vi "Flatten (single).vi"(8 "error in (no error)":errorcluster, 9 "y (0)":dbl, 10 "x (0)":dbl, 11 "XY-data":cluster{"X-array":dbl[], "Y-array":dbl[]}) -> (0 "error out":errorcluster, 3 "XY-data out":cluster{"X-array":dbl[], "Y-array":dbl[]} {"Y-array" format="%.2p"; "X-array" format="%.2p"})   [LabVIEW 2016, in "xy_utilities.lvlib"]
doc: "Add <b>x</b> to the x array of <b>XY-data</b>\nAdd <b>y</b> to the y array of <b>XY-data</b>\n\nWire data to the data input to determine the polymorphic instance to use or manually select the instance."
uses:
  xy_utilities.lvlib
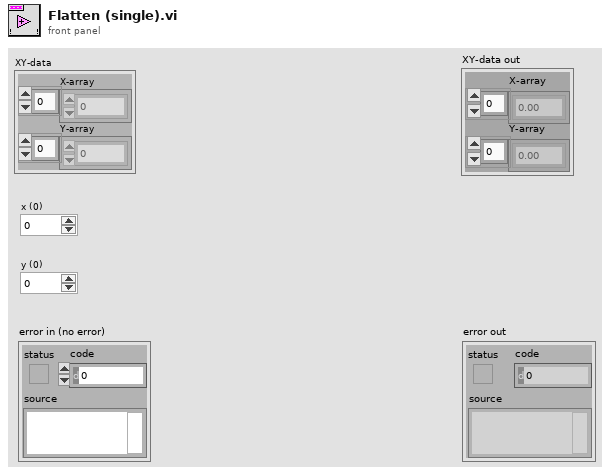
[diagram p1: front panel]
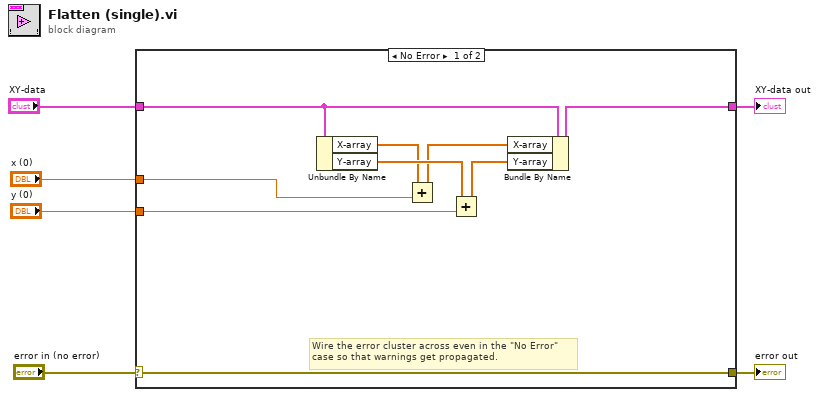
[diagram p0: block diagram]
diagram:
  n1 = case shown="No Error" "error in (no error)" {
    selector: "error in (no error)" -> [w15 w17]
    tunnel: [w15 w17] -> w5
    tunnel: "XY-data" -> [w14 w16]
    tunnel: [w13 w16] -> w3
    tunnel: "y (0)" -> [w11 _]
    tunnel: "x (0)" -> [w8 _]
    frame No Error {
      # "Wire the error cluster across even in the \"No Error\"\ncase so that warnings get propagated."
      n2 = Unbundle By Name(w14) -> ("X-array"=w9:dbl[], "Y-array"=w12:dbl[])
      n3 = Add(x=w9, y=w8) -> (x+y=w7:dbl[])
      n4 = Add(x=w12, y=w11) -> (x+y=w10:dbl[])
      n5 = Bundle By Name(cluster=w14, "X-array"=w7, "Y-array"=w10) -> (w13:cluster{"X-array":dbl[], "Y-array":dbl[]})
    }
    frame Error {
    }
  }
  "error out" <- w5
  "XY-data out" <- w3
